vi "Circuit Impedance Correction.vi"(7 "Fequency":dbl format="%#_6p", 8 "Series inductance":dbl format="%#_6p", 9 "Parallel capacitance":dbl format="%#_6p", 10 "Measured Resistance Y":dbl, 11 "Measured Resistance X":dbl) -> (1 "Calculated impedance":cdb, 2 "Corrected resistance Y":dbl, 3 "Corrected resistance X":dbl)   [LabVIEW 2016]
panel:
  in  "Sample resistance":dbl=100.0
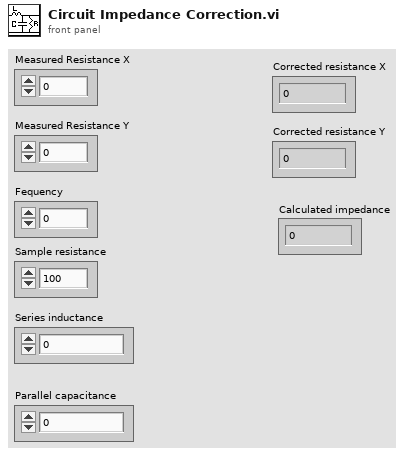
[diagram p1: front panel]
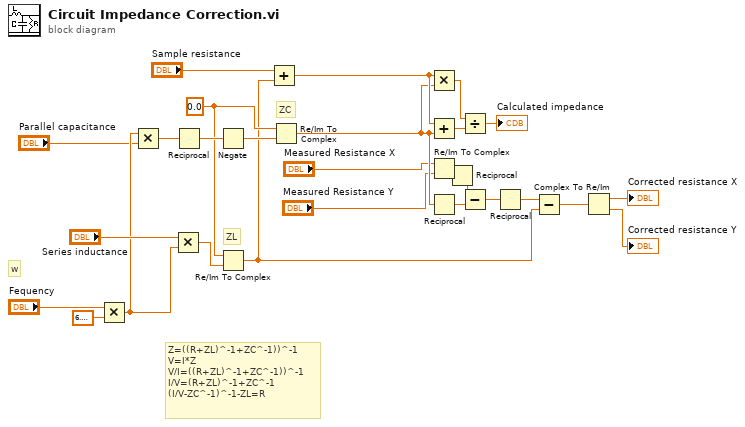
[diagram p0: block diagram]
diagram:
  w18 = 0.0 ("element")
  # "Z=((R+ZL)^-1+ZC^-1))^-1\nV=I*Z\nV/I=((R+ZL)^-1+ZC^-1))^-1\nI/V=(R+ZL)^-1+ZC^-1\n(I/V-ZC^-1)^-1-ZL=R"
  # "ZC"
  # "ZL"
  # "w"
  n1 = Multiply(x="Fequency", y=6.283185307179586) -> (x*y=w24:dbl)
  n2 = Multiply(x=w24, y="Parallel capacitance") -> (x*y=w22:dbl)
  n3 = Multiply(x="Series inductance", y=w24) -> (x*y=w19:dbl)
  n4 = Reciprocal(x=w22) -> (1/x=w21:dbl)
  n5 = Negate(x=w21) -> (-x=w20:dbl)
  n6 = Re/Im To Complex(1:w19, 2:w18) -> (0:w8:cdb)
  n7 = Add(x="Sample resistance", y=w8) -> (x+y=w14:cdb)
  n8 = Re/Im To Complex(1:w20, 2:w18) -> (0:w11:cdb)
  n9 = Multiply(x=w14, y=w11) -> (x*y=w15:cdb)
  n10 = Add(x=w14, y=w11) -> (x+y=w16:cdb)
  n11 = Re/Im To Complex(1:"Measured Resistance Y", 2:"Measured Resistance X") -> (0:w5:cdb)
  n12 = Reciprocal(x=w11) -> (1/x=w12:cdb)
  n13 = Reciprocal(x=w5) -> (1/x=w1:cdb)
  n14 = Divide(x=w15, y=w16) -> (x/y=→"Calculated impedance":cdb)
  n15 = Subtract(x=w1, y=w12) -> (x-y=w10:cdb)
  n16 = Reciprocal(x=w10) -> (1/x=w9:cdb)
  n17 = Subtract(x=w9, y=w8) -> (x-y=w3:cdb)
  n18 = Complex To Re/Im(x + iy=w3) -> (x=→"Corrected resistance X":dbl, y=→"Corrected resistance Y":dbl)
